vi "Server.vi"() -> ()   [LabVIEW 2021]
uses:
  <vilib>/MediaMongrels Ltd/WebSockets/WebSockets/WebSocket/WebSocket.lvclass/WebSocket.ctl
  <vilib>/MediaMongrels Ltd/WebSockets/WebSockets/WebSocket Server/WebSocket Server.lvclass/WebSocket Server.ctl
  <vilib>/MediaMongrels Ltd/WebSockets/WebSockets/WebSocket/Read Return Headers.vi
  <vilib>/MediaMongrels Ltd/WebSockets/WebSockets/WebSocket Server/Read Request URI.vi
  <vilib>/MediaMongrels Ltd/WebSockets/WebSockets/WebSocket Server/WebSocket Server.lvclass
  C:/Program Files (x86)/National Instruments/LabVIEW 2021/vi.lib/MediaMongrels Ltd/WebSockets/WebSockets/WebSocket/WebSocket.lvclass
  <vilib>/MediaMongrels Ltd/WebSockets/Sockets/VISA TCP Listener/VISA TCP Listener.lvclass
panel:
  in  "OK Button":bool
  in  "Path":path
  out "Request URI":string
  out "HTTP Headers":variant
  out "Received Data":string
  in  "Stop":bool
  in  "Send":bool
  in  "Data":string
  # "WebSockets Server Example"
  # "This VI is a simple example of sending/receiving data using WebSockets.\nIt waits for a single incoming WebSockets connection on Port 6123 and\nthen displays incoming string data. Strings can also be sent back to the client.\n\nInstructions for use:\n1) Run this VI\n2) Open the index.html file located in the examples folder or the 'Client Single Connection' example or deploy the 'Test Client' web service and visiting the web service URL\n3) The index.html will display the status of the connection and once established, data can be sent/received from either this VI or the index.html file.\n\nNote: For Microsoft Edge, you may need to access the index.html file by first deploying the 'Test Client' Web Service, executing \"CheckNetIsolation LoopbackExempt -a -n=Microsoft.MicrosoftEdge_8wekyb3d8bbwe\" to enable WebSockets on a loopback and then visiting http://localhost:<web service port>/index.html"
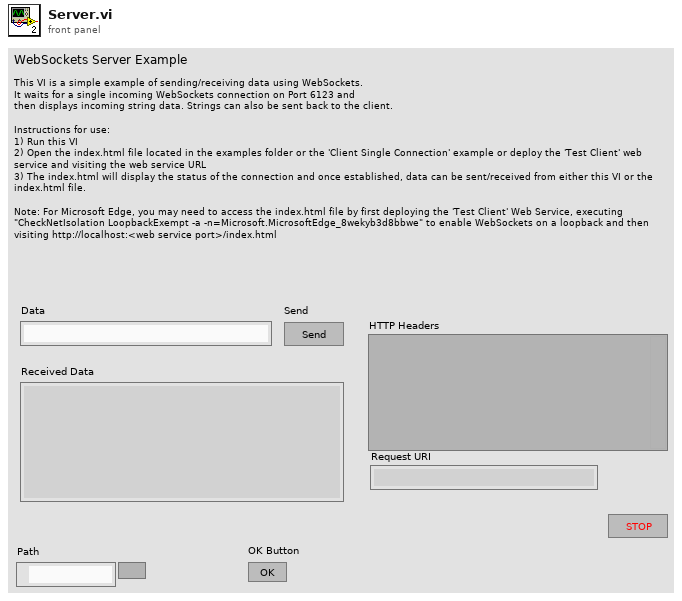
[diagram p1: front panel]
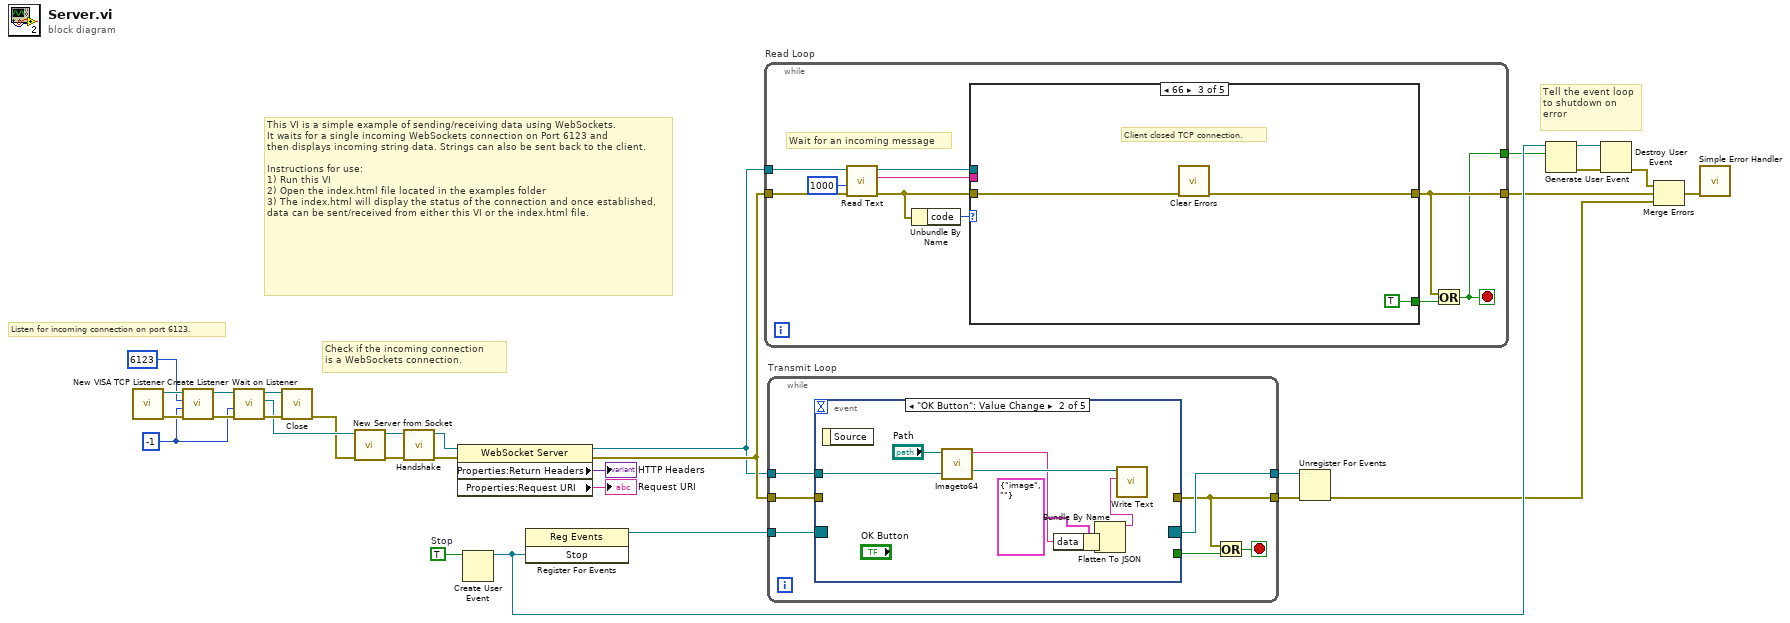
[diagram p0: block diagram]
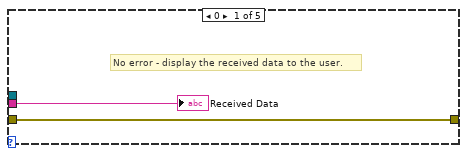
[diagram p2: hidden frame]
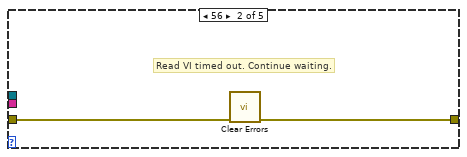
[diagram p3: hidden frame]
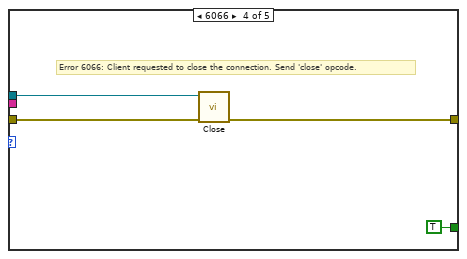
[diagram p4: hidden frame]
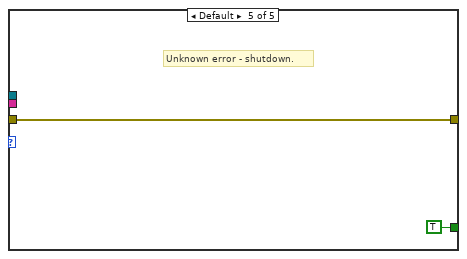
[diagram p5: hidden frame]
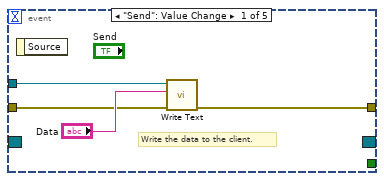
[diagram p6: hidden frame]
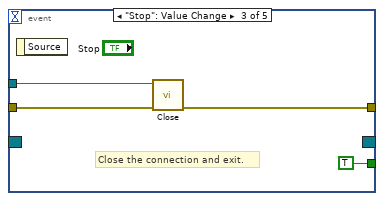
[diagram p7: hidden frame]
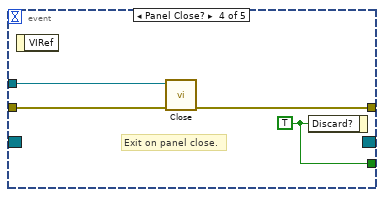
[diagram p8: hidden frame]
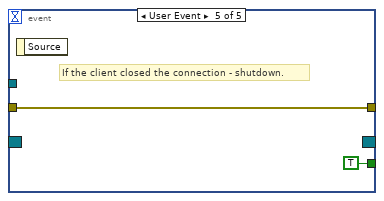
[diagram p9: hidden frame]
diagram:
  w29 = TRUE  # Stop
  w3 = -1 ("timeout ms (25000)")
  # "Tell the event loop to shutdown on error"
  # "This VI is a simple example of sending/receiving data using WebSockets.\nIt waits for a single incoming WebSockets connection on Port 6123 and\nthen displays incoming string data. Strings can also be sent back to the client.\n\nInstructions for use:\n1) Run this VI\n2) Open the index.html file located in the examples folder\n3) The index.html will display the status of the connection and once established, data can be sent/received from either this VI or the index.html file."
  # "Check if the incoming connection\nis a WebSockets connection."
  # "Listen for incoming connection on port 6123."
  n1 = call <vilib>:"New VISA TCP Listener.vi"() -> ("error out"=w9:errorcluster, "VISA TCP Listener out"=w10:refnum<class "VISA TCP Listener.lvclass">)  [unwired: 10 in]
  n2 = call-dynamic "Create Listener.vi"("error in (no error)"=w9, "timeout ms (5000)"=w3, "Port"=u16 6123 ("port"), "VISA TCP Listener in"=w10) -> ("error out"=w7:errorcluster, "VISA TCP Listener out"=w5:refnum<class "VISA TCP Listener.lvclass">)  [unwired: 6 in]
  n3 = call-dynamic "Wait on Listener.vi"("error in (no error)"=w7, "timeout ms (5000)"=w3, "VISA TCP Listener in"=w5) -> ("error out"=w8:errorcluster, "Socket out"=w2:refnum<class "Socket.lvclass">, "VISA TCP Listener out"=w6:refnum<class "VISA TCP Listener.lvclass">)  [unwired: 6 in]
  n4 = call-dynamic "Close.vi"("error in (no error)"=w8, "VISA TCP Listener in"=w6) -> ("error out"=w1:errorcluster)  [unwired: 9 in]
  n5 = call <vilib>:"New Server from Socket.vi"("error in (no error)"=w1, "Socket"=w2) -> ("error out"=w16:errorcluster, "WebSocket Server out"=w17:refnum<class "WebSocket Server.lvclass">)  [unwired: 8 in]
  n6 = call-dynamic "Handshake.vi"("error in (no error)"=w16, "WebSocket Connection in"=w17) -> ("error out"=w18:errorcluster, "WebSocket Connection out"=w14:refnum<class "WebSocket Server.lvclass">)  [unwired: 8 in]
  n7 = property class="WebSocket Server"(reference=w14, error in=w18) -> (reference out=w13:refnum<class "WebSocket Server.lvclass">, error out=w15:errorcluster, "Properties:Return Headers"=→"HTTP Headers":variant, "Properties:Request URI"=→"Request URI":string)
  n8 = Create User Event(user event datatype=w29) -> (user event=w27:refnum<user-event>)  [unwired: 1 in, 1 out]
  n9 = register-events(w27) -> (reference out=w30:refnum<event-registration>)  [unwired: 2 in, 1 out]
  n10 = while "Read Loop" {
    tunnel: w13 -> [w40]
    tunnel: [w31] -> w26
    tunnel: [w33] -> w20
    tunnel: w15 -> [w34]
    stop <- w31 stop-if-true
    # "Wait for an incoming message"
    n11 = call-dynamic "Read Text.vi"("error in (no error)"=w34, "timeout ms (5000)"=1000 ("timeout ms (25000)"), "WebSocket in"=w40) -> ("error out"=w35:errorcluster, "Data"=w37:string, "WebSocket out"=w36:refnum<class "WebSocket Server.lvclass">)  [unwired: 6 in]
    n12 = Unbundle By Name(w35) -> ("code"=w38:i32)
    n13 = case shown="66" w38 {
      tunnel: w37 -> [w42 _ _ _ _]
      tunnel: [_ _ TRUE TRUE TRUE] -> w32
      tunnel: w36 -> [_ _ _ w51 _]
      tunnel: w35 -> [w41 w44 w46 w49 w52]
      tunnel: [w41 w43 w45 w48 w52] -> w33
      frame 0 {
        # "No error - display the received data to the user."
        "Received Data" <- w42
      }
      frame 56 {
        # "Read VI timed out. Continue waiting."
        n14 = call <vilib>:"Clear Errors.vi"("error in (no error)"=w44) -> ("error out"=w43:errorcluster)  [unwired: 5 in, 1 out]
      }
      frame 66 {
        # "Client closed TCP connection."
        n15 = call <vilib>:"Clear Errors.vi"("error in (no error)"=w46) -> ("error out"=w45:errorcluster)  [unwired: 5 in, 1 out]
      }
      frame 6066 {
        # "Error 6066: Client requested to close the connection. Send 'close' opcode."
        n16 = call-dynamic "Close.vi"("error in (no error)"=w49, "WebSocket in"=w51) -> ("error out"=w48:errorcluster)  [unwired: 9 in]
      }
      frame Default {
        # "Unknown error - shutdown."
      }
    }
    n17 = Or(x=w33, y=w32) -> (x .or. y?=w31:bool)
  }
  n18 = while "Transmit Loop" {
    tunnel: w13 -> [w60]
    tunnel: w30 -> [w59]
    tunnel: [w58] -> w28
    tunnel: [w54] -> w21
    tunnel: w15 -> [w57]
    stop <- w55 stop-if-true
    n19 = event shown="[1] \"OK Button\": Value Change" {
      selector: w59 -> [_ _ _ _ _]
      dyn-events: [_ _ _ _ _] -> w58
      timeout: _ -> [_ _ _ _ _]
      tunnel: w60 -> [w64 w70 w73 w78 _]
      tunnel: [_ _ TRUE w77 TRUE] -> w56
      tunnel: [w61 _ w72 w76 w79] -> w54
      tunnel: w57 -> [w62 _ w71 w75 w79]
      event "Send": Value Change {
        # "Write the data to the client."
        n20 = event-data() -> ()  [unwired: 1 in, 1 out]
        n21 = call-dynamic "Write Text.vi"("error in (no error)"=w62, "String Data"="Data", "WebSocket in"=w64) -> ("error out"=w61:errorcluster)  [unwired: 7 in, 1 out]
      }
      event "OK Button": Value Change {
        n22 = event-data() -> ()  [unwired: 1 in, 1 out]
        n23 = call "Imageto64.vi"("path to PNG file"="Path") -> ("Base64 String"=w65:string)  [unwired: 10 in]
        n24 = Bundle By Name(cluster=cluster{"type":string, "data":string} {"type"="image", "data"=""}, "data"=w65) -> (w67:cluster{"type":string, "data":string})
        n25 = Flatten To JSON(anything=w67) -> (JSON string=w66:string)  [unwired: 2 in, 1 out]
        n26 = call-dynamic "Write Text.vi"("String Data"=w66, "WebSocket in"=w70) -> ()  [unwired: 8 in, 2 out]
      }
      event "Stop": Value Change {
        # "Close the connection and exit."
        n27 = event-data() -> ()  [unwired: 1 in, 1 out]
        n28 = call-dynamic "Close.vi"("error in (no error)"=w71, "WebSocket in"=w73) -> ("error out"=w72:errorcluster)  [unwired: 9 in]
      }
      event Panel Close? {
        w77 = TRUE ("Discard?")
        # "Exit on panel close."
        n29 = event-data() -> ()  [unwired: 1 in, 1 out]
        n30 = call-dynamic "Close.vi"("error in (no error)"=w75, "WebSocket in"=w78) -> ("error out"=w76:errorcluster)  [unwired: 9 in]
        n31 = event-data("Discard?"=w77) -> ()  [unwired: 1 in, 1 out]
      }
      event User Event {
        # "If the client closed the connection - shutdown."
        n32 = event-data() -> ()  [unwired: 1 in, 1 out]
      }
    }
    n33 = Or(x=w54, y=w56) -> (x .or. y?=w55:bool)
  }
  n34 = Unregister For Events(event registration refnum=w28, error in=w21) -> (error out=w19:errorcluster)
  n35 = Generate User Event(user event=w27, event data cluster=w26) -> (user event out=w25:refnum<user-event>, error out=w24:errorcluster)  [unwired: 2 in]
  n36 = Destroy User Event(user event=w25, error in=w24) -> (error out=w23:errorcluster)
  n37 = Merge Errors(w23, w20, w19) -> (w22:errorcluster)
  n38 = call <vilib>:"Simple Error Handler.vi"("error in (no error)"=w22) -> ()  [unwired: 4 in, 5 out]
